vi "Find Serial Type.vi"(8 "error in (no error)":errorcluster, 11 "Serial IN":string) -> (0 "error out":errorcluster, 3 "Serial Type Out":T1)   [LabVIEW 2026]
doc: "Determines serial type by using Regular Expressions (hard coded). A missing serial or a serial that does not match the pattern is Unknown.\n\nAuthored by Brad James\nbrad.james@varian.com\n\nCopyright (c) 2013, Varian Medical Systems, Inc."
uses:
  Custom Controls/Serial Type.ctl
  <vilib>/regexp/Match Regular Expression.xnode
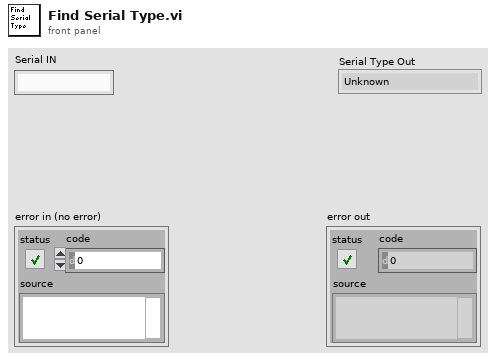
[diagram p1: front panel]
types:
  T1 = typedef "Serial Type.ctl" = enum16{"Unknown", "Tube Serial", "HE Serial", "CAP Serial"}
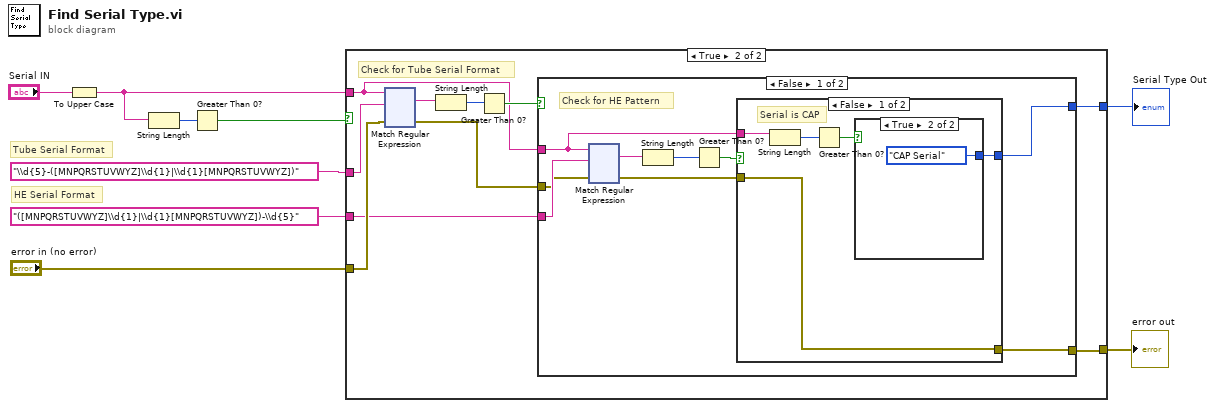
[diagram p0: block diagram]
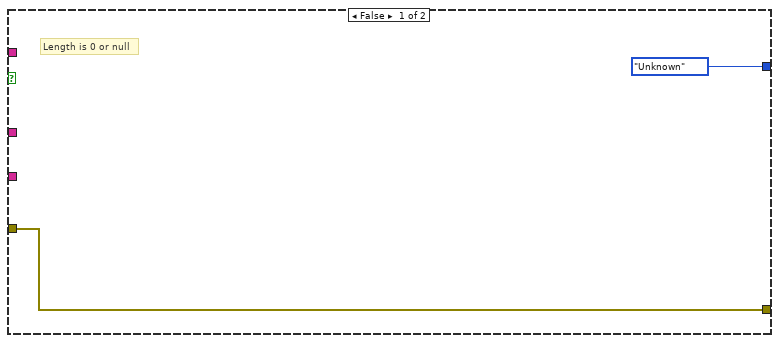
[diagram p2: hidden frame]
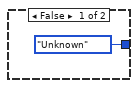
[diagram p3: hidden frame]
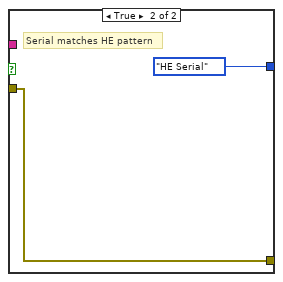
[diagram p4: hidden frame]
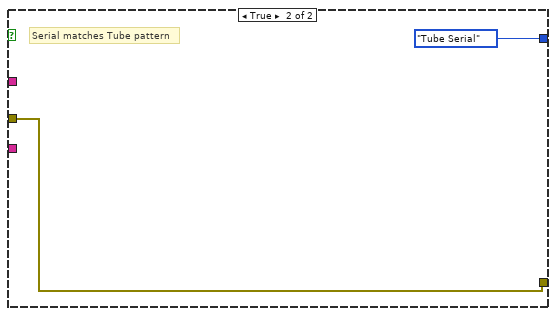
[diagram p5: hidden frame]
diagram:
  # "Tube Serial Format"
  # "HE Serial Format"
  n1 = To Upper Case(1:"Serial IN") -> (0:w6:string)
  n2 = String Length(string=w6) -> (length=w2:i32)
  n3 = Greater Than 0?(x=w2) -> (x > 0?=w1:bool)
  n4 = case shown="True" w1 {
    tunnel: "\\d{5}-([MNPQRSTUVWYZ]\\d{1}|\\d{1}[MNPQRSTUVWYZ])" -> [_ w21]
    tunnel: "([MNPQRSTUVWYZ]\\d{1}|\\d{1}[MNPQRSTUVWYZ])-\\d{5}" -> [_ w12]
    tunnel: w6 -> [_ w13]
    tunnel: [Serial_Type."Unknown" ("Serial Type Out") w16] -> w5
    tunnel: "error in (no error)" -> [w10 w20]
    tunnel: [w10 w14] -> w3
    frame False {
      # "Length is 0 or null"
    }
    frame True {
      # "Check for Tube Serial Format"
      n5 = xnode "Match Regular Expression"("input string"=w13, "regular expression"=w21, "error in"=w20) -> ("whole match"=w19:string, "error out"=w15:errorcluster)  [unwired: 3 in, 3 out]
      n6 = String Length(string=w19) -> (length=w18:i32)
      n7 = Greater Than 0?(x=w18) -> (x > 0?=w17:bool)
      n8 = case shown="False" w17 {
        tunnel: [w25 Serial_Type."Tube Serial" ("Serial Type Out")] -> w16
        tunnel: w15 -> [w29 w157]
        tunnel: [w23 w157] -> w14
        tunnel: w13 -> [w22 _]
        tunnel: w12 -> [w30 _]
        frame False {
          # "Check for HE Pattern"
          n9 = xnode "Match Regular Expression"("input string"=w22, "regular expression"=w30, "error in"=w29) -> ("whole match"=w28:string, "error out"=w24:errorcluster)  [unwired: 3 in, 3 out]
          n10 = String Length(string=w28) -> (length=w27:i32)
          n11 = Greater Than 0?(x=w27) -> (x > 0?=w26:bool)
          n12 = case shown="False" w26 {
            tunnel: [w35 Serial_Type."HE Serial" ("Serial Type Out")] -> w25
            tunnel: w24 -> [w34 w38]
            tunnel: [w34 w38] -> w23
            tunnel: w22 -> [w33 _]
            frame False {
              # "Serial is CAP"
              n13 = String Length(string=w33) -> (length=w32:i32)
              n14 = Greater Than 0?(x=w32) -> (x > 0?=w31:bool)
              n15 = case shown="True" w31 {
                tunnel: [Serial_Type."Unknown" ("Serial Type Out") Serial_Type."CAP Serial" ("Serial Type Out")] -> w35
                frame False {
                }
                frame True {
                }
              }
            }
            frame True {
              # "Serial matches HE pattern"
            }
          }
        }
        frame True {
          # "Serial matches Tube pattern"
        }
      }
    }
  }
  "Serial Type Out" <- w5
  "error out" <- w3
